vi "StringToCluster(SubVI).vi"(8 "error in (no error)":errorcluster, 10 "Проверка CRC8":bool, 11 "StringIn":string="xV4\u0012\u0002\u0000\u0000\u0000pМC\u0016њwѕa\u0000\u0000\u0001э\u0000\u0000\u0000\u0000\u0000\u0000\u0000\u0000\u0000\u0000\u0000\u0000\u0000\u0000\u0000\u0000\u0000\u0000\u0000\u0000o\u0012ѓ9\u0000\u0000\u0000\u0000\u0000\u0000\u0000\u0000+\u0019\u0000\u0000\u00002”И\u0000z\u0011") -> (0 "error out":errorcluster, 2 "CRC8Good":bool, 3 "ECC_Cluster":T1={"MagicWord"=305419896, "FrameFormatVersion"=1, "Ncycle"=1, "Reserve"=3, "GlobalTime1"=4, "GlobalTime2"=5, "Reserve2"=6, "DataSize"=7, "CRC 8"=0, "EncodersParam1"=9, "EncodersParam2"=9, "LoseSamples"=10, "SamplingInterval"=1.0, "OverloadSamplesChannelX"=11, "OverloadSamplesChannelY"=12, "Reserve3"=13, "PacketCounter"=0, "Data1"=[[0.0, 0.0, 0.0, 0.0, 0.0, 0.0, 0.8999999999068677]]} {"PacketCounter" format="%08x"; "Reserve3" format="%08x"; "OverloadSamplesChannelY" format="%04x"; "OverloadSamplesChannelX" format="%04x"; "SamplingInterval" format="%#_6e"; "LoseSamples" format="%08x"; "EncodersParam2" format="%016x"; "EncodersParam1" format="%016x"; "CRC 8" format="%02x"; "Reserve2" format="%02x"; "Reserve" format="%02x"; "Ncycle" format="%04x"; "FrameFormatVersion" format="%02x"; "MagicWord" format="%.0x"})   [LabVIEW 2017]
uses:
  Control_EU/ClusterPack (Type).ctl
panel:
  out "unsigned byte array":u8[](array[numeric]) format="%02x"
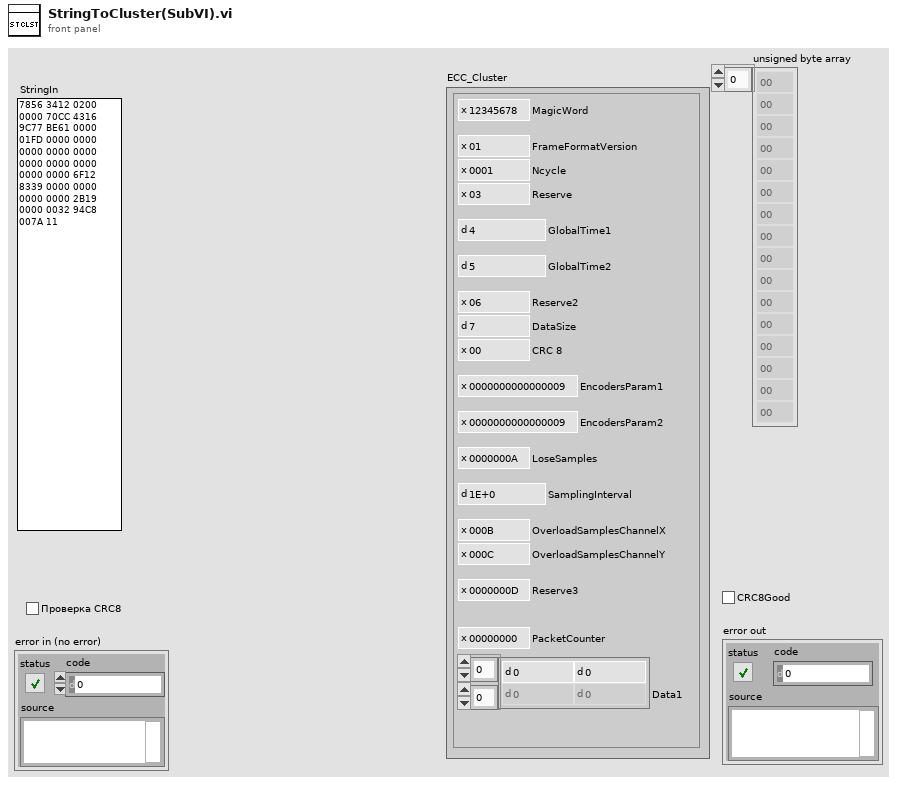
[diagram p1: front panel]
types:
  T1 = typedef "ClusterPack (Type).ctl" = cluster{"MagicWord":u32, "FrameFormatVersion":u8, "Ncycle":u16, "Reserve":u8, "GlobalTime1":u32, "GlobalTime2":u32, "Reserve2":u8, "DataSize":u16, "CRC 8":u8, "EncodersParam1":u64, "EncodersParam2":u64, "LoseSamples":u32, "SamplingInterval":sgl, "OverloadSamplesChannelX":u16, "OverloadSamplesChannelY":u16, "Reserve3":u32, "PacketCounter":u32, "Data1":dbl[][]}
  T2 = enum16{"big-endian, network order", "native, host order", "little-endian"}
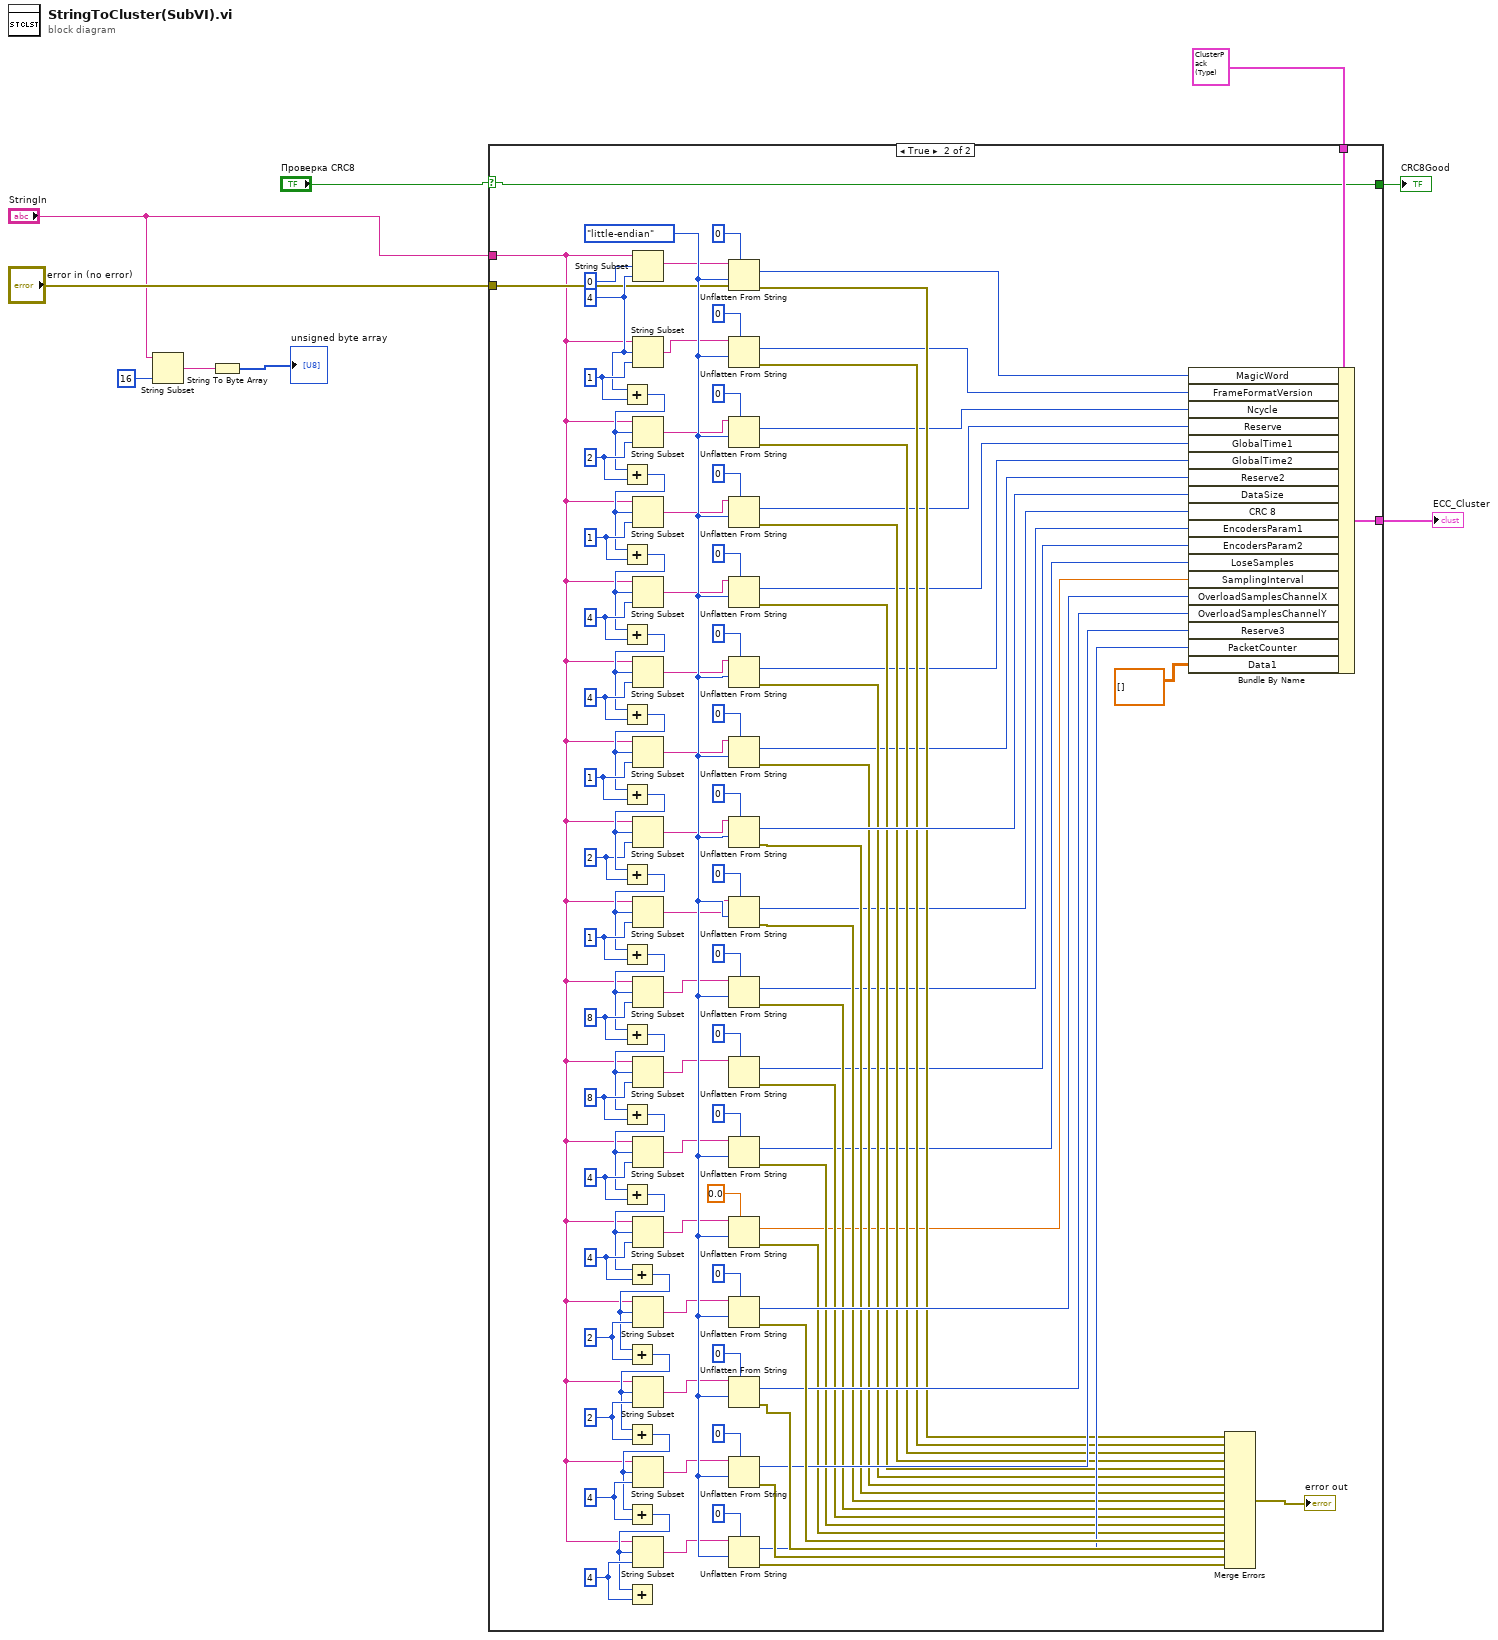
[diagram p0: block diagram]
diagram:
  n1 = String Subset(string="StringIn", length (rest)=16 ("length (rest)")) -> (substring=w4:string)  [unwired: 1 in]
  n2 = String To Byte Array(string=w4) -> (unsigned byte array=→"unsigned byte array":u8[])
  n3 = case shown="True" "Проверка CRC8" {
    selector: "Проверка CRC8" -> [w10 w12]
    tunnel: "error in (no error)" -> [_ w23]
    tunnel: T1 {"MagicWord"=305419896, "FrameFormatVersion"=1, "Ncycle"=1, "Reserve"=3, "GlobalTime1"=4, "GlobalTime2"=5, "Reserve2"=6, "DataSize"=7, "CRC 8"=0, "EncodersParam1"=9, "EncodersParam2"=9, "LoseSamples"=10, "SamplingInterval"=1.0, "OverloadSamplesChannelX"=11, "OverloadSamplesChannelY"=12, "Reserve3"=13, "PacketCounter"=0, "Data1"=[[0.0, 0.0, 0.0, 0.0, 0.0, 0.0, 0.8999999999068677]]} ("ECC_Cluster 5") -> [w11 w22]
    tunnel: [w11 w21] -> w7
    tunnel: "StringIn" -> [_ w13]
    tunnel: [w10 w12] -> w1
    frame False {
    }
    frame True {
      w117 = 4 ("length (rest)")
      w115 = 4 ("length (rest)")
      w105 = 2 ("length (rest)")
      w99 = 2 ("length (rest)")
      w97 = 4 ("length (rest)")
      w91 = 4 ("length (rest)")
      w70 = 8 ("length (rest)")
      w66 = 8 ("length (rest)")
      w59 = 1 ("length (rest)")
      w55 = 2 ("length (rest)")
      w52 = 1 ("length (rest)")
      w48 = 4 ("length (rest)")
      w119 = 4 ("length (rest)")
      w43 = 1 ("length (rest)")
      w35 = 2 ("length (rest)")
      w30 = 1 ("length (rest)")
      w108 = T2."little-endian" ("byte order (0:big-endian, network order)")
      w29 = 4 ("length (rest)")
      n4 = Add(x=w29, y=w30) -> (x+y=w34:i32)
      n5 = Add(x=w34, y=w35) -> (x+y=w38:i32)
      n6 = Add(x=w38, y=w43) -> (x+y=w42:i32)
      n7 = Add(x=w42, y=w119) -> (x+y=w47:i32)
      n8 = Add(x=w47, y=w48) -> (x+y=w51:i32)
      n9 = Add(x=w51, y=w52) -> (x+y=w57:i32)
      n10 = Add(x=w57, y=w55) -> (x+y=w58:i32)
      n11 = Add(x=w58, y=w59) -> (x+y=w65:i32)
      n12 = Add(x=w65, y=w66) -> (x+y=w69:i32)
      n13 = Add(x=w69, y=w70) -> (x+y=w73:i32)
      n14 = Add(x=w73, y=w91) -> (x+y=w90:i32)
      n15 = Add(x=w90, y=w97) -> (x+y=w98:i32)
      n16 = Add(x=w98, y=w99) -> (x+y=w104:i32)
      n17 = Add(x=w104, y=w105) -> (x+y=w114:i32)
      n18 = Add(x=w114, y=w115) -> (x+y=w116:i32)
      n19 = Add(x=w116, y=w117) -> ()  [unwired: 1 out]
      n20 = String Subset(string=w13, offset (0)=0, length (rest)=w29) -> (substring=w25:string)
      n21 = String Subset(string=w13, offset (0)=w29, length (rest)=w30) -> (substring=w28:string)
      n22 = String Subset(string=w13, offset (0)=w34, length (rest)=w35) -> (substring=w32:string)
      n23 = String Subset(string=w13, offset (0)=w38, length (rest)=w43) -> (substring=w33:string)
      n24 = String Subset(string=w13, offset (0)=w42, length (rest)=w119) -> (substring=w37:string)
      n25 = String Subset(string=w13, offset (0)=w47, length (rest)=w48) -> (substring=w41:string)
      n26 = String Subset(string=w13, offset (0)=w51, length (rest)=w52) -> (substring=w44:string)
      n27 = String Subset(string=w13, offset (0)=w57, length (rest)=w55) -> (substring=w50:string)
      n28 = String Subset(string=w13, offset (0)=w58, length (rest)=w59) -> (substring=w53:string)
      n29 = String Subset(string=w13, offset (0)=w65, length (rest)=w66) -> (substring=w61:string)
      n30 = String Subset(string=w13, offset (0)=w69, length (rest)=w70) -> (substring=w63:string)
      n31 = String Subset(string=w13, offset (0)=w73, length (rest)=w91) -> (substring=w75:string)
      n32 = String Subset(string=w13, offset (0)=w90, length (rest)=w97) -> (substring=w76:string)
      n33 = String Subset(string=w13, offset (0)=w98, length (rest)=w99) -> (substring=w93:string)
      n34 = String Subset(string=w13, offset (0)=w104, length (rest)=w105) -> (substring=w95:string)
      n35 = String Subset(string=w13, offset (0)=w114, length (rest)=w115) -> (substring=w101:string)
      n36 = String Subset(string=w13, offset (0)=w116, length (rest)=w117) -> (substring=w106:string)
      n37 = Unflatten From String(type=u32 0 ("MagicWord 2"), binary string=w25, byte order (0:big-endian, network order)=w108, error in (no error)=w23) -> (value=w19:u32, error out=w77:errorcluster)  [unwired: 1 in, 1 out]
      n38 = Unflatten From String(type=u8 0 ("MagicWord 2"), binary string=w28, byte order (0:big-endian, network order)=w108) -> (value=w18:u8, error out=w78:errorcluster)  [unwired: 2 in, 1 out]
      n39 = Unflatten From String(type=u16 0 ("MagicWord 2"), binary string=w32, byte order (0:big-endian, network order)=w108) -> (value=w17:u16, error out=w79:errorcluster)  [unwired: 2 in, 1 out]
      n40 = Unflatten From String(type=u8 0 ("MagicWord 2"), binary string=w33, byte order (0:big-endian, network order)=w108) -> (value=w16:u8, error out=w80:errorcluster)  [unwired: 2 in, 1 out]
      n41 = Unflatten From String(type=u32 0 ("MagicWord 2"), binary string=w37, byte order (0:big-endian, network order)=w108) -> (value=w15:u32, error out=w81:errorcluster)  [unwired: 2 in, 1 out]
      n42 = Unflatten From String(type=u32 0 ("MagicWord 2"), binary string=w41, byte order (0:big-endian, network order)=w108) -> (value=w14:u32, error out=w82:errorcluster)  [unwired: 2 in, 1 out]
      n43 = Unflatten From String(type=u8 0 ("MagicWord 2"), binary string=w44, byte order (0:big-endian, network order)=w108) -> (value=w46:u8, error out=w83:errorcluster)  [unwired: 2 in, 1 out]
      n44 = Unflatten From String(type=u16 0 ("MagicWord 2"), binary string=w50, byte order (0:big-endian, network order)=w108) -> (value=w120:u16, error out=w84:errorcluster)  [unwired: 2 in, 1 out]
      n45 = Unflatten From String(type=u8 0 ("MagicWord 2"), binary string=w53, byte order (0:big-endian, network order)=w108) -> (value=w56:u8, error out=w85:errorcluster)  [unwired: 2 in, 1 out]
      n46 = Unflatten From String(type=u64 0 ("MagicWord 2"), binary string=w61, byte order (0:big-endian, network order)=w108) -> (value=w62:u64, error out=w86:errorcluster)  [unwired: 2 in, 1 out]
      n47 = Unflatten From String(type=u64 0 ("MagicWord 2"), binary string=w63) -> (value=w67:u64, error out=w87:errorcluster)  [unwired: 3 in, 1 out]
      n48 = Unflatten From String(type=u32 0 ("MagicWord 2"), binary string=w75, byte order (0:big-endian, network order)=w108) -> (value=w71:u32, error out=w88:errorcluster)  [unwired: 2 in, 1 out]
      n49 = Unflatten From String(type=sgl 0.0 ("MagicWord 2"), binary string=w76, byte order (0:big-endian, network order)=w108) -> (value=w74:sgl, error out=w89:errorcluster)  [unwired: 2 in, 1 out]
      n50 = Unflatten From String(type=u16 0 ("MagicWord 2"), binary string=w93, byte order (0:big-endian, network order)=w108) -> (value=w94:u16, error out=w110:errorcluster)  [unwired: 2 in, 1 out]
      n51 = Unflatten From String(type=u16 0 ("MagicWord 2"), binary string=w95, byte order (0:big-endian, network order)=w108) -> (value=w102:u16, error out=w111:errorcluster)  [unwired: 2 in, 1 out]
      n52 = Unflatten From String(type=u32 0 ("MagicWord 2"), binary string=w101, byte order (0:big-endian, network order)=w108) -> (value=w103:u32, error out=w112:errorcluster)  [unwired: 2 in, 1 out]
      n53 = Unflatten From String(type=u32 0 ("MagicWord 2"), binary string=w106, byte order (0:big-endian, network order)=w108) -> (value=w109:u32, error out=w113:errorcluster)  [unwired: 2 in, 1 out]
      n54 = Bundle By Name(cluster=w22, "MagicWord"=w19, "FrameFormatVersion"=w18, "Ncycle"=w17, "Reserve"=w16, "GlobalTime1"=w15, "GlobalTime2"=w14, "Reserve2"=w46, "DataSize"=w120, "CRC 8"=w56, "EncodersParam1"=w62, "EncodersParam2"=w67, "LoseSamples"=w71, "SamplingInterval"=w74, "OverloadSamplesChannelX"=w94, "OverloadSamplesChannelY"=w102, "Reserve3"=w103, "PacketCounter"=w109, "Data1"=dbl[][] []) -> (w21:T1)
      n55 = Merge Errors(w77, w78, w79, w80, w81, w82, w83, w84, w85, w86, w87, w88, w89, w110, w111, w112, w113) -> (→"error out":errorcluster)
    }
  }
  "ECC_Cluster" <- w7
  "CRC8Good" <- w1
